vi "Add Error.vi"(0 "Error Interface In":refnum<class "Error Interface.lvclass">, 1 "Error":T1, 5 "error in (no error)":errorcluster) -> (14 "Error Interface Out":refnum<class "Error Interface.lvclass">, 19 "error out":errorcluster)   [LabVIEW 2019, in "Error Interface.lvclass"]
uses:
  Error Interface.lvclass
  ErrorEvent.ctl
  Error Interface.lvclass/Error Interface.ctl
  Application.lvclass
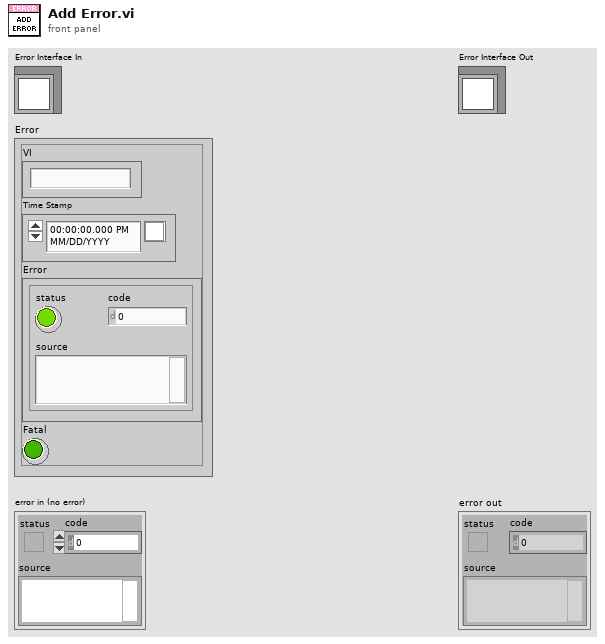
[diagram p1: front panel]
types:
  T1 = typedef "Application.lvclass/ErrorEvent.ctl" = cluster{"VI":string, "Time Stamp":timestamp, "Error":errorcluster, "Fatal":bool}
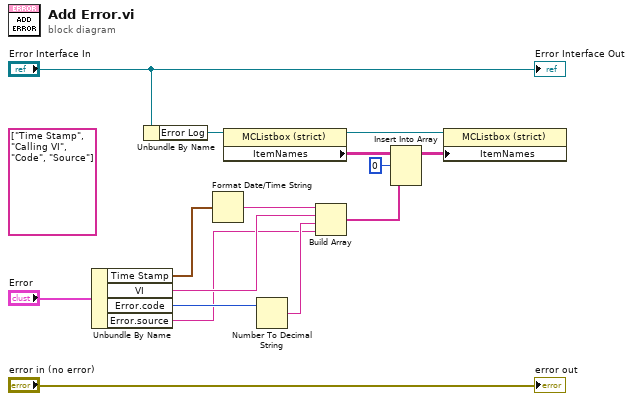
[diagram p0: block diagram]
diagram:
  (unwired) string[] ["Time Stamp", "Calling VI", "Code", "Source"] ("Column Header Strings[]")
  n1 = Unbundle By Name("Error") -> ("Time Stamp"=w8:timestamp, "VI"=w4:string, "Error.code"=w3:i32, "Error.source"=w1:string)
  n2 = Unbundle By Name("Error Interface In") -> ("Error Log"=w12:refnum<vi>)
  n3 = Format Date/Time String(seconds (now)=w8) -> (date/time string=w7:string)  [unwired: 2 in]
  n4 = property class="MCListbox (strict)"(reference=w12) -> (reference out=w10:refnum<vi>, "ItemNames"=w11:string[][])  [unwired: 1 in, 1 out]
  n5 = Number To Decimal String(number=w3) -> (decimal integer string=w2:string)  [unwired: 1 in]
  n6 = Build Array(w7, w4, w2, w1) -> (w6:string[])
  n7 = Insert Into Array(array=w11, index (row)=0, new element=w6) -> (w9:string[][])  [unwired: 1 in]
  n8 = property class="MCListbox (strict)"(reference=w10, "ItemNames"=w9) -> ()  [unwired: 1 in, 2 out]
  "error out" <- "error in (no error)"
  "Error Interface Out" <- "Error Interface In"
